vi "Tree Glyphs.vi"() -> (2 "Demo Glyph Index":i32, 3 "Folder Glyph Index":i32)   [LabVIEW 2020]
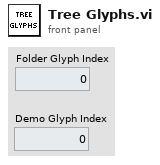
[diagram p1: front panel]
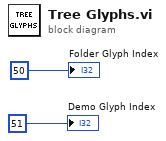
[diagram p0: block diagram]
diagram:
  "Folder Glyph Index" <- 50 ("Index")
  "Demo Glyph Index" <- 51 ("Demo Glyph Index")
